vi "PIDAutoTune_Step_Execute.vi"(5 "Procedure Type":enum16{"Open Loop Step", "Closed Loop Step"}(ring), 7 "Configuration Parameters":T2={"Controller Constant Type"=enum."Ziegler Nicols - Normal", "Type of Controller"=enum."PI", "CO Offset"=0.25, "Kn"=1.0, "Tuning Tolerance"=0.001, "Plant Tolerance"=0.001, "Newest Avg Time "=1, "Long Ave Time"=6}, 8 "Sampling Time dt (s)":dbl=0.02, 9 "Tune":bool, 10 "Measurement  (PV)":dbl, 11 "Control Output (Co)":dbl) -> (0 "Plant and Test Data":T4, 1 "New Tuning Parameters":T3, 2 "Tuning Done":bool, 3 "Adj CO":dbl, 4 "Error Occured":bool, 6 "Diagnostic Info":T1)   [LabVIEW 2019, in "Trajectory_Library.lvlib"]
doc: "This routine can be used to make a step change to a PID control loop, track the results, and calculate PID tuning parameters. It wraps the NI LabVIEW PID auto-tuning functions for use with the WPILIB LabVIEW Math PID. \n\nWarning -- This routine will modify the control output. Use it in such a manner to be able to stop the tuning if problems occur -- like running out of field space while tuning a drive motor. \n\nInputs:\n -- Procedure Type -- enum -- The type of tuning procedure to be used: Values are:\n -- Open Loop Step -- This uses the frozen CO input when the test starts. A step change is made to the output. This is the recommended method\n -- Closed Loop Step -- This uses the continually changing CO input and adds an offset value to this during the test. \n\n -- Configuration Parameters -- cluster -- This contains the parameters defining the conditions of the test. Use the Pack routine to create this data cluster.\n -- Control Output -- double -- The Control Output (CO) value from the output of the PID to be tuned.\n -- Measurement (PV) -- double -- The Process Variable (PV) value used by the PID to be tuned.\n -- Tune -- boolean -- When TRUE, tuning is performed..\n -- Sampling time -- double -- Loop time in seconds. How fast the PID and this autotune function are executed. (Optional: Default 0.02 seconds) \n\nOutputs:\n -- Adj CO -- double -- The adjusted CO. This is sent to the actuator. (This vi is put between the PID and the actuator device)\n -- Tuning Done -- boolean -- This is set to TRUE when tuning has completed. Depending on the PV noise, tuning may never be \"DONE\". However if the new tuning parameters are relatively constant, they can still be used.\n -- New Tuning Parameters -- cluster --- Data cluster containing the calculated PID tuning parameters. \n -- Plant and Test Data -- cluster -- Data cluster containing information describing the transfer function of the system being controlled (Plant).\n -- Error Occured -- Boolean -- If TRUE, an error occured.\n -- Diagnostic Info -- cluster -- This contains additional information about the test being perfromed."
uses:
  Trajectory_Library.lvlib
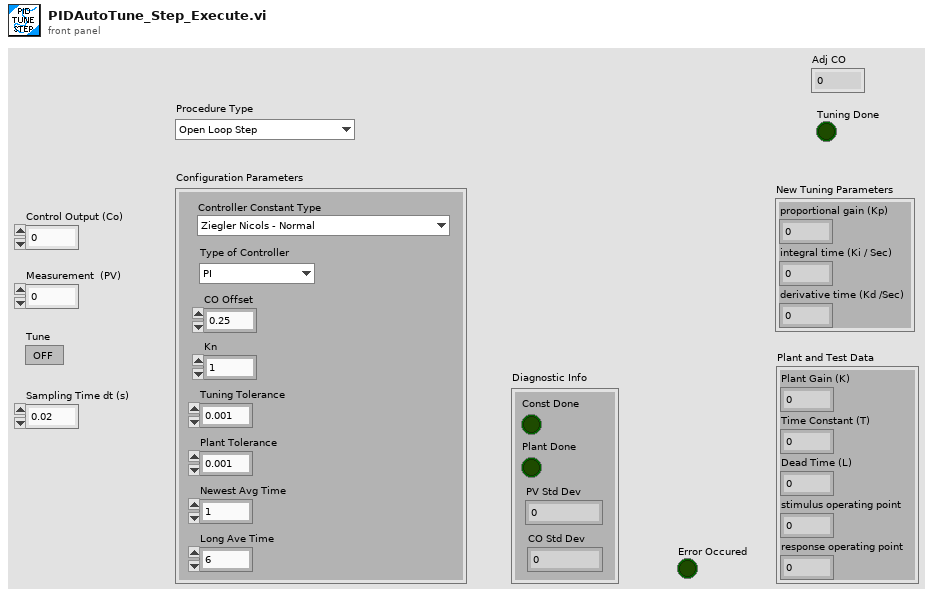
[diagram p1: front panel]
types:
  T1 = cluster{"Const Done":bool, "Plant Done":bool, "PV Std Dev":dbl, "CO Std Dev":dbl}
  T2 = cluster{"Controller Constant Type":enum16{"Ziegler Nicols - Fast", "Ziegler Nicols - Normal", "Ziegler Nicols - Slow", "CHR regulator - 0% overshoot", "CHR regulator - 20% overshoot", "CHR servo - 0 % overshoot", "CHR servo - 20% overshoot"}, "Type of Controller":enum16{"P", "PI", "PID"}, "CO Offset":dbl, "Kn":dbl, "Tuning Tolerance":dbl, "Plant Tolerance":dbl, "Newest Avg Time ":i32, "Long Ave Time":i32}
  T3 = cluster{"proportional gain (Kp)":dbl, "integral time (Ki / Sec)":dbl, "derivative time (Kd /Sec)":dbl}
  T4 = cluster{"Plant Gain (K)":dbl, "Time Constant (T)":dbl, "Dead Time (L)":dbl, "stimulus operating point":dbl, "response operating point":dbl}
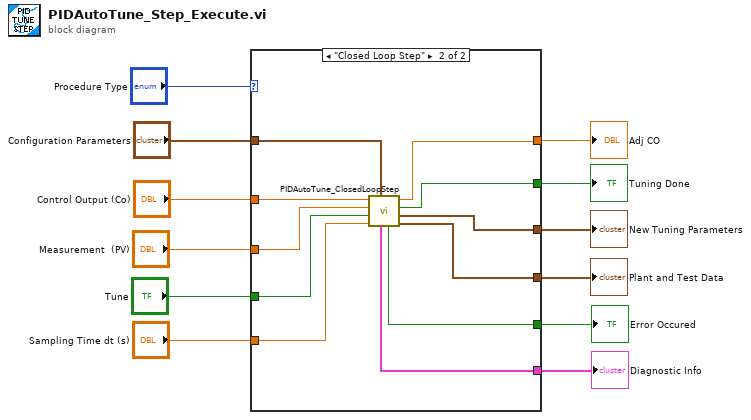
[diagram p0: block diagram]
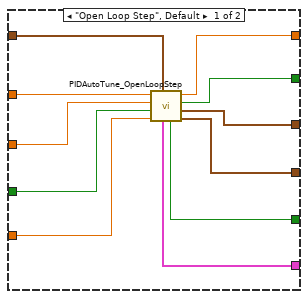
[diagram p2: hidden frame]
diagram:
  n1 = case shown="\"Closed Loop Step\"" "Procedure Type" {
    tunnel: "Configuration Parameters" -> [w23 w34]
    tunnel: "Control Output (Co)" -> [w22 w33]
    tunnel: "Measurement  (PV)" -> [w21 w32]
    tunnel: "Tune" -> [w20 w31]
    tunnel: "Sampling Time dt (s)" -> [w19 w30]
    tunnel: [w18 w29] -> w6
    tunnel: [w17 w28] -> w5
    tunnel: [w16 w27] -> w4
    tunnel: [w15 w26] -> w3
    tunnel: [w14 w25] -> w2
    tunnel: [w13 w24] -> w1
    frame "Open Loop Step", Default {
      n2 = call "PIDAutoTune_OpenLoopStep.vi"("Configuration Parameters"=w23, "Sampling Time dt (s)"=w19, "Tune"=w20, "Measurement  (PV)"=w21, "Control Output (Co)"=w22) -> ("Plant and Test Data"=w15:T4, "New Tuning Parameters"=w16:T3, "Tuning Done"=w17:bool, "Adj CO"=w18:dbl, "Error Occured"=w14:bool, "Diagnostic"=w13:T1)  [unwired: 1 in]
    }
    frame "Closed Loop Step" {
      n3 = call "PIDAutoTune_ClosedLoopStep.vi"("Configuration Parameters"=w34, "Sampling Time dt (s)"=w30, "Tune"=w31, "Measurement  (PV)"=w32, "Control Output (Co)"=w33) -> ("Plant and Test Data"=w26:T4, "New Tuning Parameters"=w27:T3, "Tuning Done"=w28:bool, "Adj CO"=w29:dbl, "Error Occured"=w25:bool, "Diagnostic"=w24:T1)  [unwired: 1 in]
    }
  }
  "Plant and Test Data" <- w3
  "Tuning Done" <- w5
  "Adj CO" <- w6
  "New Tuning Parameters" <- w4
  "Error Occured" <- w2
  "Diagnostic Info" <- w1
